vi "Configure Waveform Logging.vi"(8 "error in (no error)":errorcluster, 9 "dt":dbl, 10 "Log Waveforms":bool, 11 "Triggered Log in":refnum<class "Triggered Log.lvclass">) -> (0 "error out":errorcluster, 3 "Triggered Log out":refnum<class "Triggered Log.lvclass">)   [LabVIEW 2012, in "Triggered Log.lvclass"]
uses:
  Triggered Log.lvclass
  Triggered Log.lvclass/Triggered Log.ctl
  Shared/Classes/Log File Specifications/TDMS Log File Specification/TDMS Log File Specification.lvclass
  Engine/Classes/Logs/Segmented Logs/Segmented Log/Segmented Log.lvclass/Segmented Log.ctl
  Engine/Classes/Logs/Segmented Logs/Segmented Log/Segmented Log.lvclass
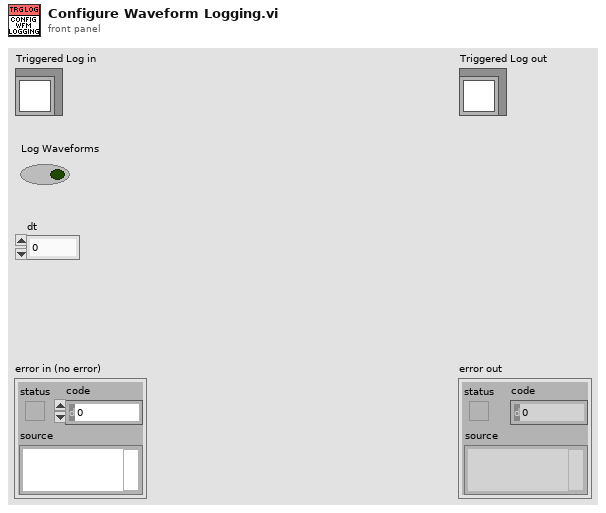
[diagram p1: front panel]
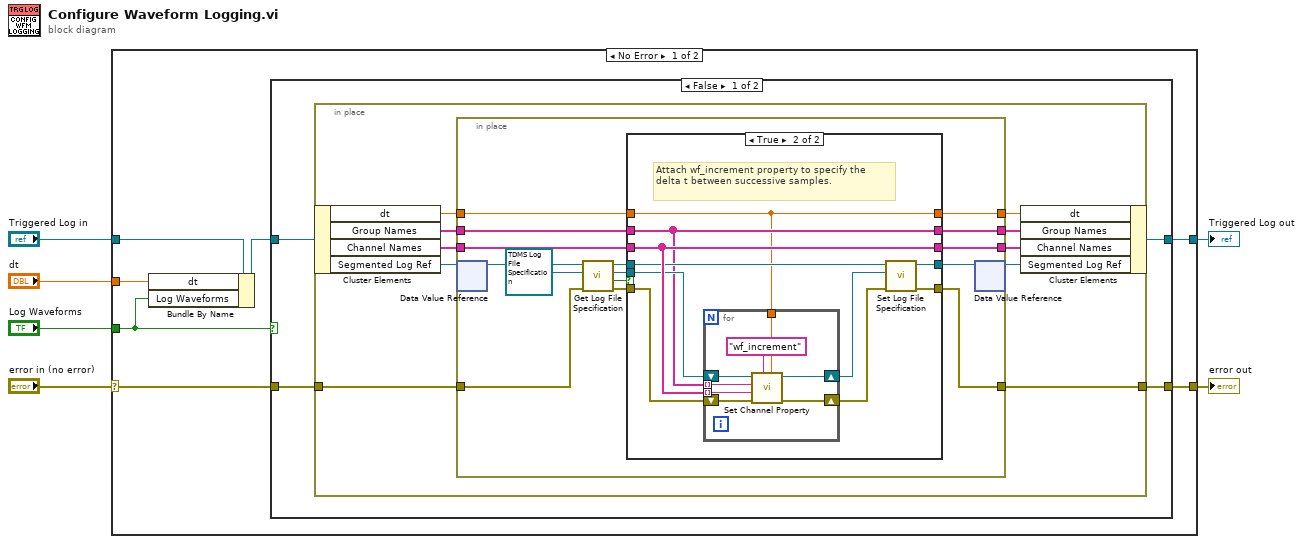
[diagram p0: block diagram]
diagram:
  n1 = case shown="No Error" "error in (no error)" {
    selector: "error in (no error)" -> [w7 w69]
    tunnel: "Triggered Log in" -> [w13 w68]
    tunnel: [w10 w68] -> w5
    tunnel: "dt" -> [w12 _]
    tunnel: "Log Waveforms" -> [w11 _]
    tunnel: [w8 w69] -> w1
    frame No Error {
      n2 = Bundle By Name(cluster=w13, "dt"=w12, "Log Waveforms"=w11) -> (w9:refnum<class "Triggered Log.lvclass">)
      n3 = case shown="False" w11 {
        tunnel: [w16 w66] -> w10
        tunnel: w9 -> [w17 w66]
        tunnel: [w15 w67] -> w8
        tunnel: w7 -> [w14 w67]
        frame False {
          n4 = in-place {
            in-place-border: [w25] -> w15
            in-place-border: w14 -> [w24]
            n5 = in-place-cluster #1(w17) -> ("dt"=w18:dbl, "Group Names"=w23:string[], "Channel Names"=w22:string[], "Segmented Log Ref"=w27:refnum<data-value>)
            n6 = in-place {
              in-place-border: [w37] -> w25
              in-place-border: w24 -> [w39]
              in-place-border: w23 -> [w36]
              in-place-border: w22 -> [w35]
              in-place-border: [w34] -> w21
              in-place-border: [w33] -> w20
              in-place-border: [w32] -> w19
              in-place-border: w18 -> [w31]
              n7 = in-place-dvr #2(w27) -> (w41:refnum<class "Segmented Log.lvclass">)  [unwired: 1 out]
              n8 = call "Get Log File Specification.vi"("error in (no error)"=w39, "Log File Specification type"=refnum<class "TDMS Log File Specification.lvclass"> refnum ("TDMS Log File Specification.lvclass"), "Segmented Log in"=w41) -> ("error out"=w42:errorcluster, "Is expected type?"=w28:bool, "Log File Specification"=w29:refnum<class "TDMS Log File Specification.lvclass">, "Segmented Log out"=w40:refnum<class "Segmented Log.lvclass">)  [unwired: 5 in]
              n9 = case shown="True" w28 {
                tunnel: w40 -> [w47 w56]
                tunnel: [w47 w55] -> w38
                tunnel: [w46 w54] -> w37
                tunnel: w29 -> [_ w52]
                tunnel: w42 -> [w46 w53]
                tunnel: w36 -> [w44 w51]
                tunnel: w35 -> [w43 w57]
                tunnel: [w44 w51] -> w34
                tunnel: [w43 w57] -> w33
                tunnel: [w45 w50] -> w32
                tunnel: w31 -> [w45 w50]
                frame False {
                  # "No need to attach timing metadata properties to non-TDMS files"
                }
                frame True {
                  # "Attach wf_increment property to specify the delta t between successive samples."
                  n10 = for {
                    shift-right: [w58] -> w48
                    shift-left: w52 -> [w64]
                    shift-right: [w59] -> w49
                    shift-left: w53 -> [w65]
                    tunnel: w51 -> [w63] mode=indexing
                    tunnel: w57 -> [w62] mode=indexing
                    tunnel: w50 -> [w60]
                    n11 = call "Set Channel Property.vi"("Value"=w60, "Name"="wf_increment", "error in (no error)"=w65, "Channel Name in"=w62, "Group Name in"=w63, "TDMS Log File Specification in"=w64) -> ("error out"=w59:errorcluster, "TDMS Log File Specification out"=w58:refnum<class "TDMS Log File Specification.lvclass">)  [unwired: 2 in, 2 out]
                  }
                  n12 = call "Set Log File Specification.vi"("error in (no error)"=w49, "Log File Specification.lvclass"=w48, "Segmented Log in"=w56) -> ("error out"=w54:errorcluster, "Segmented Log out"=w55:refnum<class "Segmented Log.lvclass">)  [unwired: 7 in]
                }
              }
              n13 = in-place-dvr #2(w38) -> (w26:refnum<data-value>)  [unwired: 1 out]
            }
            n14 = in-place-cluster #1("dt"=w19, "Group Names"=w21, "Channel Names"=w20, "Segmented Log Ref"=w26) -> (w16:refnum<class "Triggered Log.lvclass">)
          }
        }
        frame True {
          # "Timing properties will automatically be tagged if log files are written with waveform data."
        }
      }
    }
    frame Error {
    }
  }
  "error out" <- w1
  "Triggered Log out" <- w5
